vi "Implement Authenticate.vi"(8 "error in":errorcluster, 10 "Challenge Dict":string, 11 "WampCraaAuthenticator in":refnum<class "WampCraAuthenticator.lvclass">) -> (0 "error out":errorcluster, 1 "Authenticate Dict":string, 2 "Authenticate Signature":string, 3 "WampCraaAuthenticator out":refnum<class "WampCraAuthenticator.lvclass">)   [LabVIEW 2020, in "wamplv.lvlib" / "WampCraAuthenticator.lvclass"]
uses:
  WampCraAuthenticator.lvclass
  PBKDF2 hash type.ctl
  WampCraAuthenticator.lvclass/WampCraAuthenticator.ctl
  0c520959-8ddd-4bdc-a188-1738126c2762.vi
  87c86cf2-f7c8-4f8a-85be-5d546ab5bd99.vi
  351a13fb-45f8-4654-b200-6ac5ad740662.vi
  13e31f3d-cf19-4c16-a000-bd40e0710092.vi
  <vilib>/JDP Science/JSONtext/Find Item.vi
  Utils/Base64 Encode.vi
  <vilib>/JDP Science/JSONtext/Next JSON Value.vi
  <vilib>/JDP Science/JSONtext/String Subset.vi
  <vilib>/JDP Science/JSONtext/Parsing/Advance past next JSON Value (inlined COPY).vi
  <vilib>/JDP Science/JSONtext/Parsing/Advance past whitespace.vi
  <vilib>/JDP Science/JSONtext/Parsing/Advance past String.vi
  <vilib>/JDP Science/JSONtext/Parsing/Advance past Number.vi
  <vilib>/JDP Science/JSONtext/Parsing/Advance past Line Ending.vi
  <vilib>/JDP Science/JSONtext/Parsing/Parse Full Path or Item Name.vi
  <vilib>/JDP Science/JSONtext/Parsing/Advance past Array.vi
  <vilib>/JDP Science/JSONtext/Parsing/Advance past Object.vi
  <vilib>/JDP Science/JSONtext/support/Error Cluster From Code.vi
  <vilib>/JDP Science/JSONtext/Offset/Find Item Locations by Path.vi
  <vilib>/JDP Science/JSONtext/JSON text to Variant.vi
  <vilib>/JDP Science/JSONtext/LVClass Serializer/JSONtext LVClass Serializer.lvclass
  Utils/Utils.lvclass
  HashLib/HashLib.lvclass
  wamplv.lvlib
panel:
  in  "PBKDF2 hash type":T1
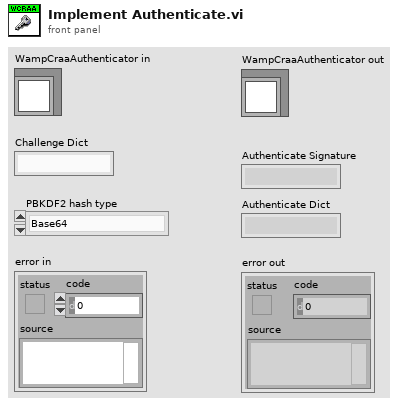
[diagram p1: front panel]
types:
  T1 = typedef "wamplv.lvlib/PBKDF2 hash type.ctl" = enum8{"Base64", "Hex string, lower case", "Hex string, upper case", "Direct to string cast"}
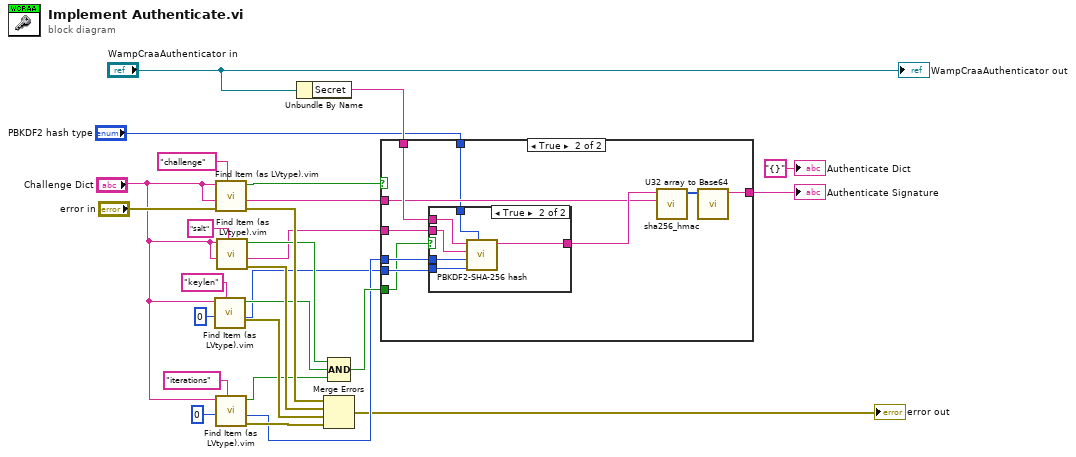
[diagram p0: block diagram]
diagram:
  n1 = call "Find Item (as LVtype).vim"("$Path or Item Name"="keylen", "Data Type and Default Value"=0, "JSON"="Challenge Dict") -> ("error out"=w11:errorcluster, "Data"=w4:i32, "Found"=w8:bool)  [unwired: 5 in, 1 out]
  n2 = call "Find Item (as LVtype).vim"("$Path or Item Name"="challenge", "error in (no error)"="error in", "Data Type and Default Value"="Challenge Dict", "JSON"="Challenge Dict") -> ("error out"=w13:errorcluster, "Data"=w20:string, "Found"=w21:bool)  [unwired: 4 in, 1 out]
  n3 = call "Find Item (as LVtype).vim"("$Path or Item Name"="iterations", "Data Type and Default Value"=0, "JSON"="Challenge Dict") -> ("error out"=w10:errorcluster, "Data"=w5:i32, "Found"=w2:bool)  [unwired: 5 in, 1 out]
  n4 = call "Find Item (as LVtype).vim"("$Path or Item Name"="salt", "Data Type and Default Value"="Challenge Dict", "JSON"="Challenge Dict") -> ("error out"=w12:errorcluster, "Data"=w6:string, "Found"=w9:bool)  [unwired: 5 in, 1 out]
  n5 = Unbundle By Name("WampCraaAuthenticator in") -> ("Secret"=w26:string)
  n6 = Merge Errors(w13, w12, w11, w10) -> (→"error out":errorcluster)
  n7 = Compound Arithmetic op=AND(w9, w8, w2) -> (w7:bool)
  n8 = case shown="True" w21 {
    tunnel: w26 -> [_ w37]
    tunnel: [_ w33] -> w24
    tunnel: w20 -> [_ w29]
    tunnel: w7 -> [_ w32]
    tunnel: w6 -> [_ w36]
    tunnel: w5 -> [_ w35]
    tunnel: w4 -> [_ w34]
    tunnel: "PBKDF2 hash type" -> [_ w28]
    frame False {
    }
    frame True {
      n9 = case shown="True" w32 {
        tunnel: w37 -> [w38 w43]
        tunnel: w36 -> [_ w42]
        tunnel: w35 -> [_ w41]
        tunnel: w34 -> [_ w40]
        tunnel: [w38 w44] -> w30
        tunnel: w28 -> [_ w39]
        frame False {
        }
        frame True {
          n10 = call "PBKDF2-SHA-256 hash.vi"("PBKDF2 hash type"=w39, "Key Length"=w40, "Iterations"=w41, "Salt"=w42, "Secret"=w43) -> ("Hash string"=w44:string)  [unwired: 6 in]
        }
      }
      n11 = call "sha256_hmac.vi"("data"=w29, "key"=w30) -> ("sha256"=w31:u32[])  [unwired: 9 in]
      n12 = call "U32 array to Base64.vi"("Array"=w31) -> ("Base64 sring out"=w33:string)  [unwired: 10 in]
    }
  }
  "Authenticate Signature" <- w24
  "WampCraaAuthenticator out" <- "WampCraaAuthenticator in"
  "Authenticate Dict" <- "{}" ("Authenticate Dict")
